vi "Match End.vi"(8 "error in (no error)":errorcluster, 11 "Alpaca JSON Parser in":refnum<class "JSON Parser.lvclass">) -> (0 "error out":errorcluster, 3 "Alpaca JSON Parser out":refnum<class "JSON Parser.lvclass">)   [LabVIEW 2019, in "JKI JSON Serialization.lvlib" / "JSON Parser.lvclass"]
doc: "JKI Serialization 1.0.0.11\nTomi Maila - JKI\nCopyright (c) 2016, JKI\n\nJKI JSON 1.1.10.37\nTomi Maila - JKI\nCopyright (c) 2017, JKI"
uses:
  JSON Parser.lvclass
  JSON Lexer/JSON Token Type.ctl
  JSON Lexer/JSON Lexer.lvclass
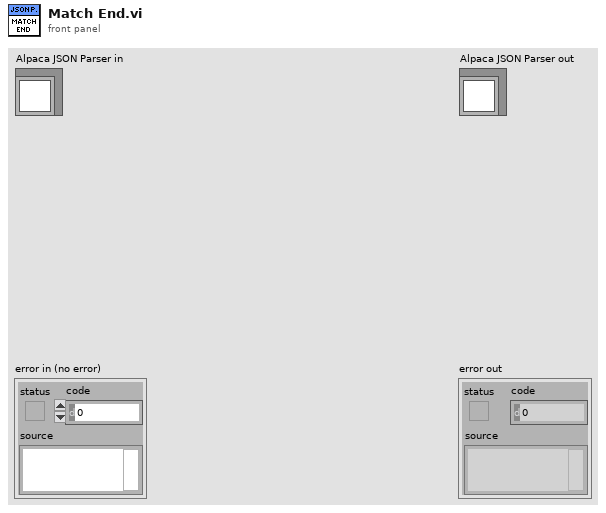
[diagram p1: front panel]
types:
  T1 = typedef "JKI JSON Serialization.lvlib/JSON Lexer.lvclass/JSON Token Type.ctl" = enum32{"unknown", "comma", "end-label", "begin-object", "end-object", "begin-array", "end-array", "quoted-string", "boolean", "exponential-number", "decimal-number", "integer-number", "special-number", "null", "symbol", "whitespace", "EOF"}
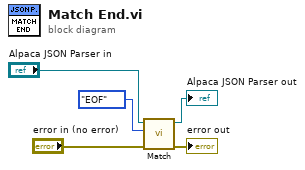
[diagram p0: block diagram]
diagram:
  n1 = call-dynamic "Match.vi"("error in (no error)"="error in (no error)", "Token Type"=JSON_Token_Type."EOF" ("JSON Token Type"), "Alpaca Parser in"="Alpaca JSON Parser in") -> ("error out"=→"error out":errorcluster, "Alpaca Parser out"=→"Alpaca JSON Parser out":refnum<class "JSON Parser.lvclass">)  [unwired: 7 in]
